vi "areaOfTriangle.vi"() -> ()   [LabVIEW 2025]
doc: "Calculates the area of a triangle using the base and height provided as inputs"
panel:
  out "area of triangle":dbl
  in  "height":dbl
  in  "base":dbl
  # "Calculate area of triangle"
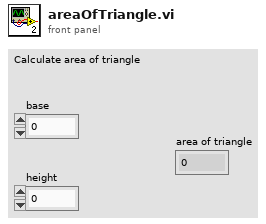
[diagram p1: front panel]
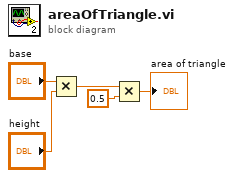
[diagram p0: block diagram]
diagram:
  n1 = Multiply(x="base", y="height") -> (x*y=w3:dbl)
  n2 = Multiply(x=w3, y=0.5) -> (x*y=→"area of triangle":dbl)
